vi "get available modules to pair.vi"(8 "error in":errorcluster, 11 "editor in":refnum<data-value>) -> (0 "error out":errorcluster, 1 "Display Name":string[](array[string]), 2 "IDs":string[](array[string]), 3 "editor out":refnum<data-value>)   [LabVIEW 2013, in "TEC editor node.lvclass"]
uses:
  TEC editor node.lvclass
  module/configuration/TEC configuration.lvclass
  <vilib>/NI/Configuration Framework/serializable configuration/NISE_CEF_serializable configuration.lvclass/NISE_CEF_serializable configuration.ctl
  <vilib>/NI/Configuration Framework/serializable configuration/NISE_CEF_serializable configuration.lvclass
  <vilib>/NI/Configuration Framework/serializable configuration/Read UID.vi
  read pair information.vi
  <vilib>/NI/Tag Bus Data Framework/Configuration Editor/Classes/Module editor node/Read display name.vi
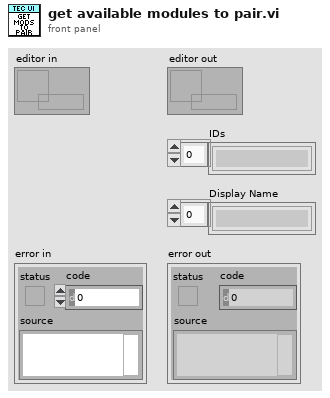
[diagram p1: front panel]
types:
  T1 = typedef "TEC editor node.lvclass/pair information.ctl" = cluster{"paired guid":string}
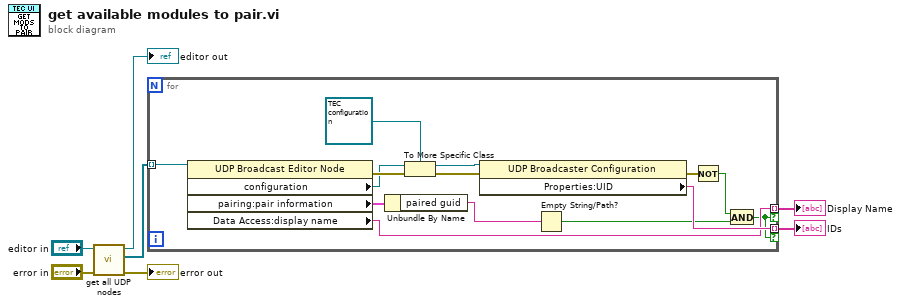
[diagram p0: block diagram]
diagram:
  n1 = call "get all UDP nodes.vi"("error in"="error in", "editor in"="editor in") -> ("error out"=→"error out":errorcluster, "All UDP refs"=w1:refnum<data-value>[], "editor out"=→"editor out":refnum<data-value>)  [unwired: 7 in]
  n2 = for {
    tunnel: w1 -> [w21] mode=indexing
    tunnel: [w19] -> w7 mode=indexing if=w8
    tunnel: [w9] -> w6 mode=indexing if=w8
    n3 = property class="UDP Broadcast Editor Node"(reference=w21) -> (error out=w20:errorcluster, "configuration"=w15:refnum<class "NISE_CEF_serializable configuration.lvclass">, "pairing:pair information"=w12:T1, "Data Access:display name"=w9:string)  [unwired: 1 in, 1 out]
    n4 = Unbundle By Name(w12) -> ("paired guid"=w11:string)
    n5 = To More Specific Class(target class=refnum<class "TEC configuration.lvclass"> refnum ("UDP Broadcaster Configuration"), reference=w15, error in=w20) -> (specific class reference=w14:refnum<class "TEC configuration.lvclass">, error out=w16:errorcluster)
    n6 = property class="UDP Broadcaster Configuration"(reference=w14, error in=w16) -> (error out=w18:errorcluster, "Properties:UID"=w19:string)  [unwired: 1 out]
    n7 = Empty String/Path?(string/path=w11) -> (empty?=w10:bool)
    n8 = Not(x=w18) -> (.not. x?=w17:bool)
    n9 = And(x=w17, y=w10) -> (x .and. y?=w8:bool)
  }
  "IDs" <- w7
  "Display Name" <- w6
